vi "TextToVariant.vi"(7 "Data Type":variant, 8 "error in (no error)":errorcluster, 10 "Serializable Text":string, 11 "BlueSerializer in":refnum<class "BlueSerializer.lvclass">) -> (0 "error out":errorcluster, 2 "Variant out":variant, 3 "BlueSerializer out":refnum<class "BlueSerializer.lvclass">)   [LabVIEW 2020, in "BlueSerialization.lvlib" / "BlueSerializer.lvclass"]
uses:
  BlueSerializer.lvclass
  <vilib>/Utility/error.llb/Error Cluster From Error Code.vi
  <vilib>/ErrorRing/Error Ring.xnode
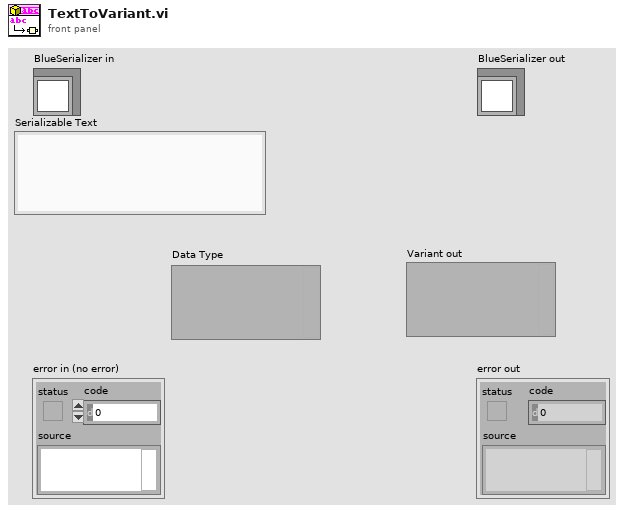
[diagram p1: front panel]
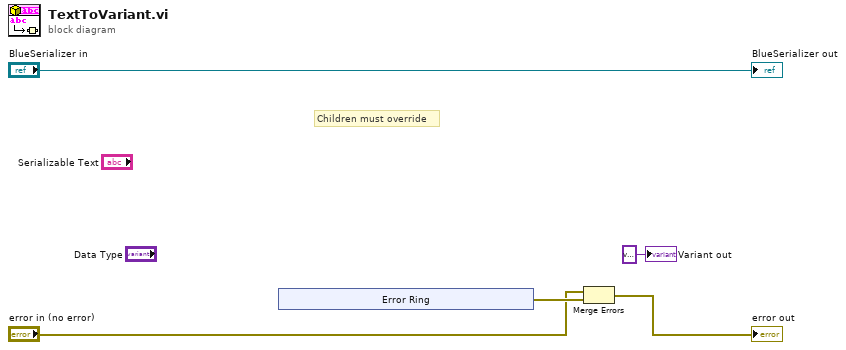
[diagram p0: block diagram]
diagram:
  # "Children must override"
  n1 = xnode "Error Ring"() -> ("error out"=w4:errorcluster)
  n2 = Merge Errors("error in (no error)", w4) -> (→"error out":errorcluster)
  "BlueSerializer out" <- "BlueSerializer in"
  "Variant out" <- variant ("Variant out")
